vi "Panel-AlignRasterAO.vi"() -> ()   [LabVIEW 2009]
uses:
  <vilib>/Analysis/Matrix/Datatypes/RealMatrix.ctl
  <vilib>/Analysis/baseanly.llb/A x Vector.vi
  <vilib>/Analysis/Matrix/Numeric/Multiply/Multiply - RM,R.vi
  <vilib>/Analysis/NI_AALBase.lvlib
  <vilib>/Analysis/Matrix/NI_Matrix.lvlib
panel:
  out "Collecting Data":bool
  in  "RESET":bool
  in  "ALIGN":bool
  out "XY Graph":cluster{dbl[], dbl[]}(graph)
  in  "STOP":bool
  in  "AO":enum16{"K1", "K2"}(ring)
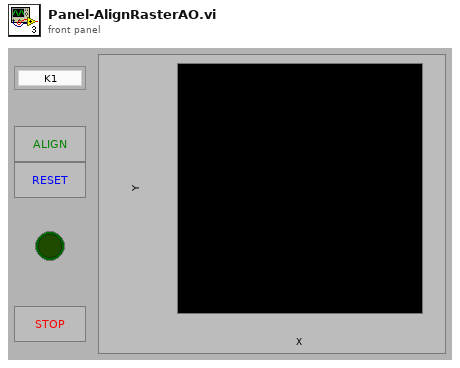
[diagram p1: front panel]
types:
  T1 = typedef "NI_Matrix.lvlib/RealMatrix.ctl" = dbl[][]
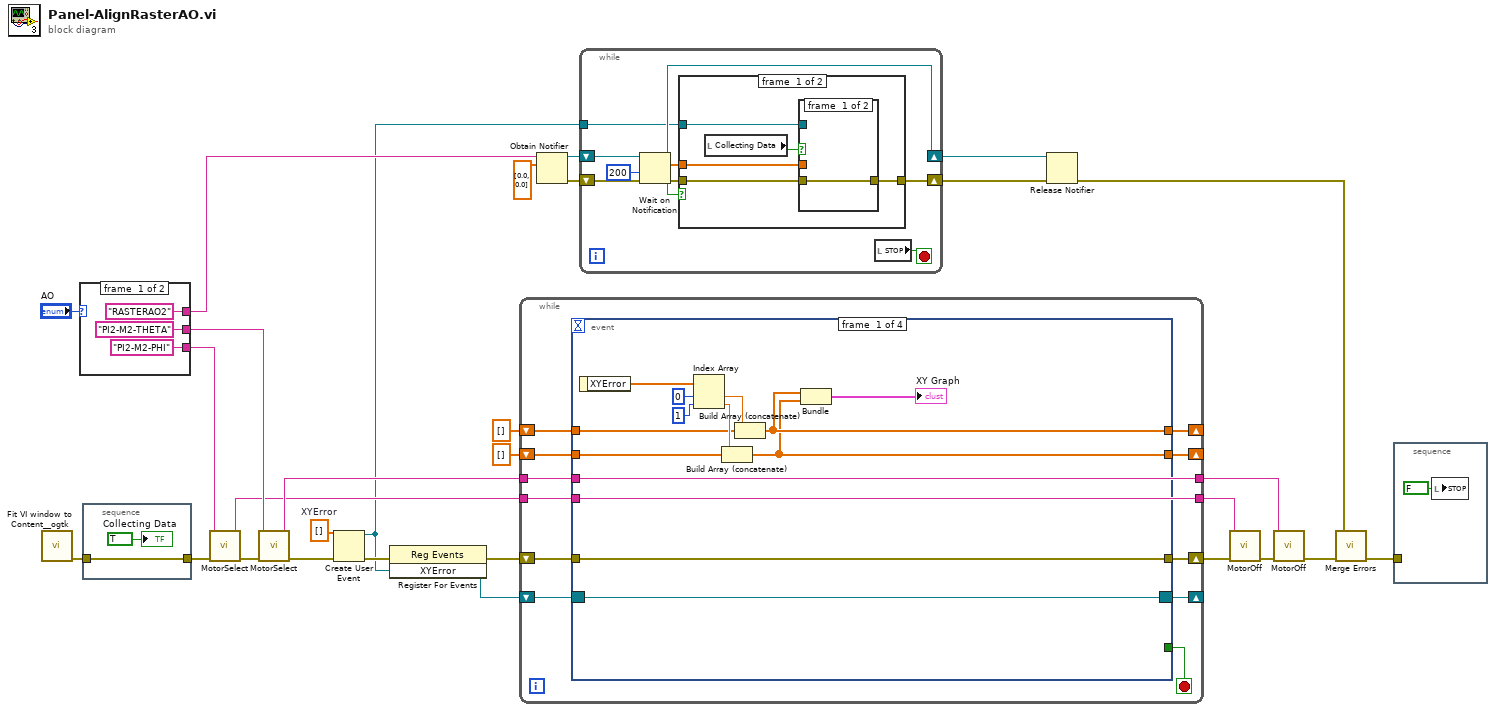
[diagram p0: block diagram]
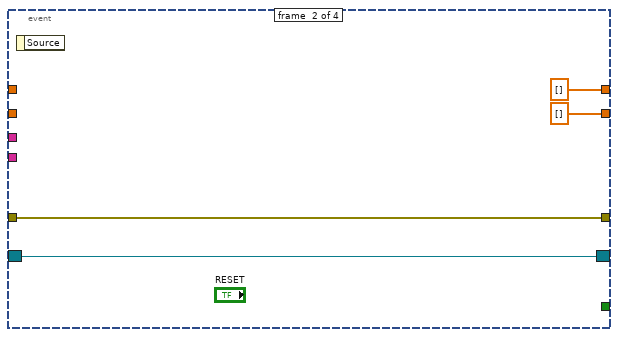
[diagram p2: hidden frame]
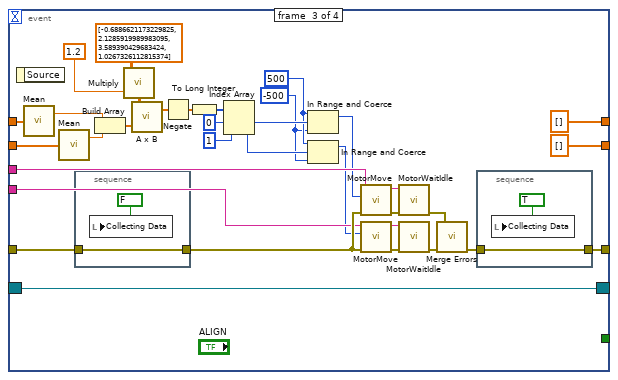
[diagram p3: hidden frame]
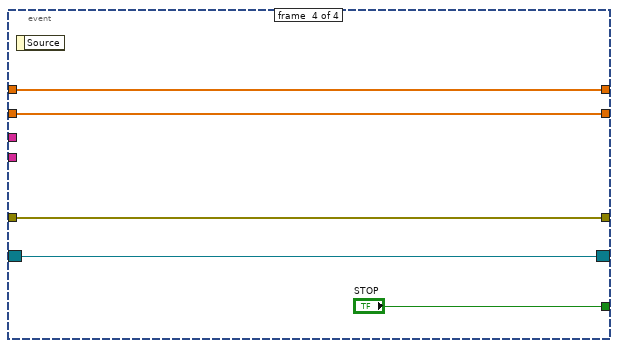
[diagram p4: hidden frame]
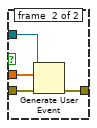
[diagram p5: hidden frame]
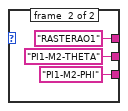
[diagram p7: hidden frame]
diagram:
  w21 = dbl[] []  # XYError
  n1 = call <userlib>:"Fit VI window to Content__ogtk.vi"() -> ("error out"=w1:errorcluster)  [unwired: 3 in, 4 out]
  n2 = case shown="\"K2\"" "AO" {
    tunnel: ["RASTERAO2" "RASTERAO1"] -> w11
    tunnel: ["PI2-M2-THETA" "PI1-M2-THETA"] -> w24
    tunnel: ["PI2-M2-PHI" "PI1-M2-PHI"] -> w23
    frame #0 {
    }
    frame #1 {
    }
  }
  n3 = stacked-sequence {
    tunnel: [w36] -> w2
    tunnel: w1 -> [w36]
    frame #0 {
      "Collecting Data" <- TRUE ("Collecting Data")
    }
  }
  n4 = call "MotorSelect.vi"("Motor"=w23, "error in (no error)"=w2) -> ("Motor out"=w12:string, "error out"=w17:errorcluster)  [unwired: 6 out]
  n5 = call "MotorSelect.vi"("Motor"=w24, "error in (no error)"=w17) -> ("Motor out"=w13:string, "error out"=w16:errorcluster)  [unwired: 6 out]
  n6 = Create User Event(user event datatype=w21, error in=w16) -> (user event=w6:refnum<user-event>, error out=w20:errorcluster)
  n7 = register-events(error in=w20, w6) -> (reference out=w18:refnum<event-registration>, error out=w19:errorcluster)  [unwired: 1 in]
  n8 = while {
    shift-right: [w41] -> w10
    shift-left: w19 -> [w48]
    shift-right: [w46] -> _
    shift-left: w18 -> [w47]
    shift-right: [w44] -> _
    shift-left: dbl[] [] -> [w45]
    shift-right: [w42] -> _
    shift-left: dbl[] [] -> [w43]
    tunnel: w12 -> [w39]
    tunnel: w13 -> [w40]
    tunnel: [w40] -> w7
    tunnel: [w39] -> w9
    stop <- w38 stop-if-true
    n9 = event shown="[2] \"ALIGN\": Value Change" {
      selector: w47 -> [w49 w62 w79 w103]
      dyn-events: [w49 w62 w79 w103] -> w46
      timeout: _ -> [_ _ _ _]
      tunnel: w48 -> [w50 w61 w78 w106]
      tunnel: w45 -> [w54 _ w83 w105]
      tunnel: [w53 dbl[] [] dbl[] [] w105] -> w44
      tunnel: w43 -> [w52 _ w82 w104]
      tunnel: [w51 dbl[] [] dbl[] [] w104] -> w42
      tunnel: [w50 w61 w75 w106] -> w41
      tunnel: w40 -> [_ _ w74 _]
      tunnel: w39 -> [_ _ w73 _]
      tunnel: [_ _ _ "STOP"] -> w38
      event #0 {
        n10 = event-data() -> ("XYError"=w55:dbl[])  [unwired: 1 out]
        n11 = Index Array(array=w55, index #1=0 ("index"), index #2=1 ("index")) -> (element #1=w59:dbl, element #2=w58:dbl)
        n12 = Build Array (concatenate)(w52, w58) -> (w51:dbl[])
        n13 = Build Array (concatenate)(w54, w59) -> (w53:dbl[])
        n14 = Bundle(w53, w51) -> (→"XY Graph":cluster{dbl[], dbl[]})  [unwired: 1 out]
      }
      event #1 {
        n15 = event-data() -> ()  [unwired: 2 out]
      }
      event #2 {
        w65 = -500 ("lower limit")
        w66 = 500 ("upper limit")
        n16 = event-data() -> ()  [unwired: 2 out]
        n17 = call <vilib>:"Mean.vi"("X"=w83) -> ("mean"=w96:dbl)  [unwired: 1 out]
        n18 = call <vilib>:"Mean.vi"("X"=w82) -> ("mean"=w97:dbl)  [unwired: 1 out]
        n19 = stacked-sequence {
          tunnel: w78 -> [w102]
          tunnel: [w102] -> w77
          frame #0 {
            n20 = local write "Collecting Data"(FALSE ("Collecting Data")) -> ()
          }
        }
        n21 = Build Array(w96, w97) -> (w98:dbl[])
        n22 = call-poly <vilib>:"Multiply.vi"("Real Scalar c"=1.2, "Real Matrix A"=T1 [[-0.6886621173229825, 2.1285919989983095], [3.589390429683424, 1.0267326112815374]] ("Inverse Matrix 2")) -> ("A * c"=w72:T1)
        n23 = call-poly <vilib>:"A x B.vi"("Vector"=w98, "A"=w72) -> ("A x Vector"=w86:dbl[])  [unwired: 1 out]
        n24 = Negate(x=w86) -> (-x=w88:dbl[])
        n25 = To Long Integer(number=w88) -> (32bit integer=w89:i32[])
        n26 = Index Array(array=w89, index #1=0 ("index"), index #2=1 ("index")) -> (element #1=w70:i32, element #2=w68:i32)
        n27 = In Range and Coerce(upper limit=w66, x=w70, lower limit=w65) -> (coerced(x)=w69:i32)  [unwired: 1 out]
        n28 = In Range and Coerce(upper limit=w66, x=w68, lower limit=w65) -> (coerced(x)=w67:i32)  [unwired: 1 out]
        n29 = call "MotorMove.vi"("Motor"=w74, "Movement"=w69, "error in (no error)"=w77) -> ("Motor out"=w93:string, "error out"=w92:errorcluster)  [unwired: 5 out]
        n30 = call "MotorMove.vi"("Motor"=w73, "Movement"=w67, "error in (no error)"=w77) -> ("Motor out"=w95:string, "error out"=w94:errorcluster)  [unwired: 5 out]
        n31 = call "MotorWaitIdle.vi"("Motor"=w93, "error in (no error)"=w92) -> ("error out"=w84:errorcluster)  [unwired: 7 out]
        n32 = call "MotorWaitIdle.vi"("Motor"=w95, "error in (no error)"=w94) -> ("error out"=w85:errorcluster)  [unwired: 7 out]
        n33 = call <vilib>:"Merge Errors.vi"("error in 3 (no error)"=w85, "error in 2 (no error)"=w84) -> ("error out"=w76:errorcluster)  [unwired: 2 in, 3 out]
        n34 = stacked-sequence {
          tunnel: w76 -> [w100]
          tunnel: [w100] -> w75
          frame #0 {
            n35 = local write "Collecting Data"(TRUE ("Collecting Data")) -> ()
          }
        }
      }
      event #3 {
        n36 = event-data() -> ()  [unwired: 2 out]
      }
    }
  }
  n37 = Obtain Notifier(name (unnamed)=w11, notification data type=dbl[] [0.0, 0.0]) -> (notifier out=w22:refnum<notifier>, error out=w27:errorcluster)  [unwired: 2 in, 1 out]
  n38 = while {
    shift-right: [w115] -> w26
    shift-left: w22 -> [w117]
    shift-right: [w109] -> w25
    shift-left: w27 -> [w116]
    tunnel: w6 -> [w113]
    stop <- w108 stop-if-true
    n39 = Wait on Notification(notifier=w117, timeout in ms (-1)=200, error in (no error)=w116) -> (notifier out=w115:refnum<notifier>, notification=w112:dbl[], timed out?=w110:bool, error out=w114:errorcluster)  [unwired: 1 out]
    n40 = case shown="False" w110 {
      tunnel: w114 -> [w122 w128]
      tunnel: w113 -> [w121 _]
      tunnel: w112 -> [w120 _]
      tunnel: [w119 w128] -> w109
      frame #0 {
        n41 = local read "Collecting Data"() -> (w118:bool)
        n42 = case shown="True" w118 {
          tunnel: w122 -> [w123 w127]
          tunnel: w121 -> [_ w126]
          tunnel: w120 -> [_ w125]
          tunnel: [w123 w124] -> w119
          frame #0 {
          }
          frame #1 {
            n43 = Generate User Event(user event=w126, event data cluster=w125, error in=w127) -> (error out=w124:errorcluster)  [unwired: 1 out]
          }
        }
      }
      frame #1 {
      }
    }
    n44 = local read "STOP"() -> (w108:bool)
  }
  n45 = Release Notifier(notifier=w26, error in (no error)=w25) -> (error out=w4:errorcluster)  [unwired: 3 out]
  n46 = call "MotorOff.vi"("Motor"=w9, "error in (no error)"=w10) -> ("error out"=w8:errorcluster)  [unwired: 7 out]
  n47 = call "MotorOff.vi"("Motor"=w7, "error in (no error)"=w8) -> ("error out"=w5:errorcluster)  [unwired: 7 out]
  n48 = call <vilib>:"Merge Errors.vi"("error in 3 (no error)"=w5, "error in 2 (no error)"=w4) -> ("error out"=w3:errorcluster)  [unwired: 2 in, 3 out]
  n49 = stacked-sequence {
    tunnel: w3 -> [_]
    frame #0 {
      n50 = local write "STOP"(FALSE ("STOP")) -> ()
    }
  }
